vi "measureEcho.vi"() -> ()   [LabVIEW 2016]
uses:
  <vilib>/Utility/file.llb/Write Delimited Spreadsheet (DBL).vi
panel:
  in  "AFC & OFC Measurement time":i32=2
  in  "Burn time/ RFC measurement time":i32=2
  in  "Cluster":T1={"span"=300000000.0, "rbw"=10000.0, "enableVBW"=FALSE, "vbw"=0.0, "traceLength"=64001, "window"=0, "verticalUnit"=0, "center freq"=150000000.0} {"verticalUnit" items=["SpectrumVerticalUnit_dBm", "SpectrumVerticalUnit_Watt", "SpectrumVerticalUnit_Volt", "SpectrumVerticalUnit_Amp", "SpectrumVerticalUnit_dBmV"]; "window" items=["SpectrumWindow_Kaiser", "SpectrumWindow_Mil6dB", "SpectrumWindow_BlackmanHarris", "SpectrumWindow_Rectangle", "SpectrumWindow_FlatTop", "SpectrumWindow_Hann"]; "traceLength" items=["801"=801, "2401"=2401, "4001"=4001, "8001"=8001, "10401"=10401, "16001"=16001, "32001"=32001, "64001"=64001]}
  out "Duration array":T2(array[cluster])
  in  "Array":T3(array[cluster])=[{"Enable ASF?"=TRUE, "Channel Frequency (MHz)"=80.0, "ASF"=0.185, "Enable Frequency Sweep"=FALSE, "Sweep Parameters"={"Start Frequency (MHz)"=80.5, "Stop Frequency (MHz)"=89.25, "Rising Step Size (MHz)"=0.04375, "Falling Step Size (MHz)"=0.0, "Falling Step Interval (ms)"=0.01, "Rising Step Interval (ms)"=1.0}, "Rising/Falling"=FALSE}, {"Enable ASF?"=TRUE, "Channel Frequency (MHz)"=110.0, "ASF"=0.185, "Enable Frequency Sweep"=TRUE, "Sweep Parameters"={"Start Frequency (MHz)"=70.0, "Stop Frequency (MHz)"=160.0, "Rising Step Size (MHz)"=0.0006, "Falling Step Size (MHz)"=0.0, "Falling Step Interval (ms)"=0.01, "Rising Step Interval (ms)"=1.0}, "Rising/Falling"=FALSE}, {"Enable ASF?"=FALSE, "Channel Frequency (MHz)"=80.0, "ASF"=0.1, "Enable Frequency Sweep"=FALSE, "Sweep Parameters"={"Start Frequency (MHz)"=80.5, "Stop Frequency (MHz)"=89.25, "Rising Step Size (MHz)"=0.04375, "Falling Step Size (MHz)"=0.0, "Falling Step Interval (ms)"=0.01, "Rising Step Interval (ms)"=1.0}, "Rising/Falling"=FALSE}, {"Enable ASF?"=TRUE, "Channel Frequency (MHz)"=80.0, "ASF"=0.1, "Enable Frequency Sweep"=TRUE, "Sweep Parameters"={"Start Frequency (MHz)"=40.0, "Stop Frequency (MHz)"=115.0, "Rising Step Size (MHz)"=0.0006, "Falling Step Size (MHz)"=0.0, "Falling Step Interval (ms)"=0.01, "Rising Step Interval (ms)"=1.0}, "Rising/Falling"=FALSE}] {"Sweep Parameters"."Rising Step Interval (ms)" min=0.0 max=2.55 step=0.01 format="%.4f"; "Sweep Parameters"."Stop Frequency (MHz)" min=0.0 max=400.0 step=1.0 format="%.6f"; "Sweep Parameters"."Start Frequency (MHz)" min=0.0 max=400.0 step=1.0 format="%.6f"; "Sweep Parameters"."Falling Step Interval (ms)" min=0.0 max=2.55 step=0.01 format="%.2f"; "Sweep Parameters"."Falling Step Size (MHz)" min=0.0 max=400.0 step=0.1 format="%.6f"; "Sweep Parameters"."Rising Step Size (MHz)" min=0.0 max=400.0 step=0.1 format="%.7f"; "ASF" min=0.0 max=1.0 step=0.001 format="%.3f"; "Channel Frequency (MHz)" min=0.0 max=400.0 step=1.0 format="%.6f"}
  in  "Folder for all data (Don't forget the last slash!)":string="C:\\Users\\Lab\\Desktop\\Data\\2019-08\\2019-08-07\\"
  out "Inst. Freq":dbl=1000000.0
  in  "Shuffle?":bool
  in  "Start freq":dbl=1000000.0 format="%0.2e"
  in  "End freq":dbl=2000000.0 format="%0.2e"
  in  "Freq step":i32=100000 format="%.2e"
  out "error out":errorcluster
  in  "error in":errorcluster
  in  "Mod shape":enum16{"Triangle", "Sine"}(ring)
  # "RSA settings"
  # "Modulation settings"
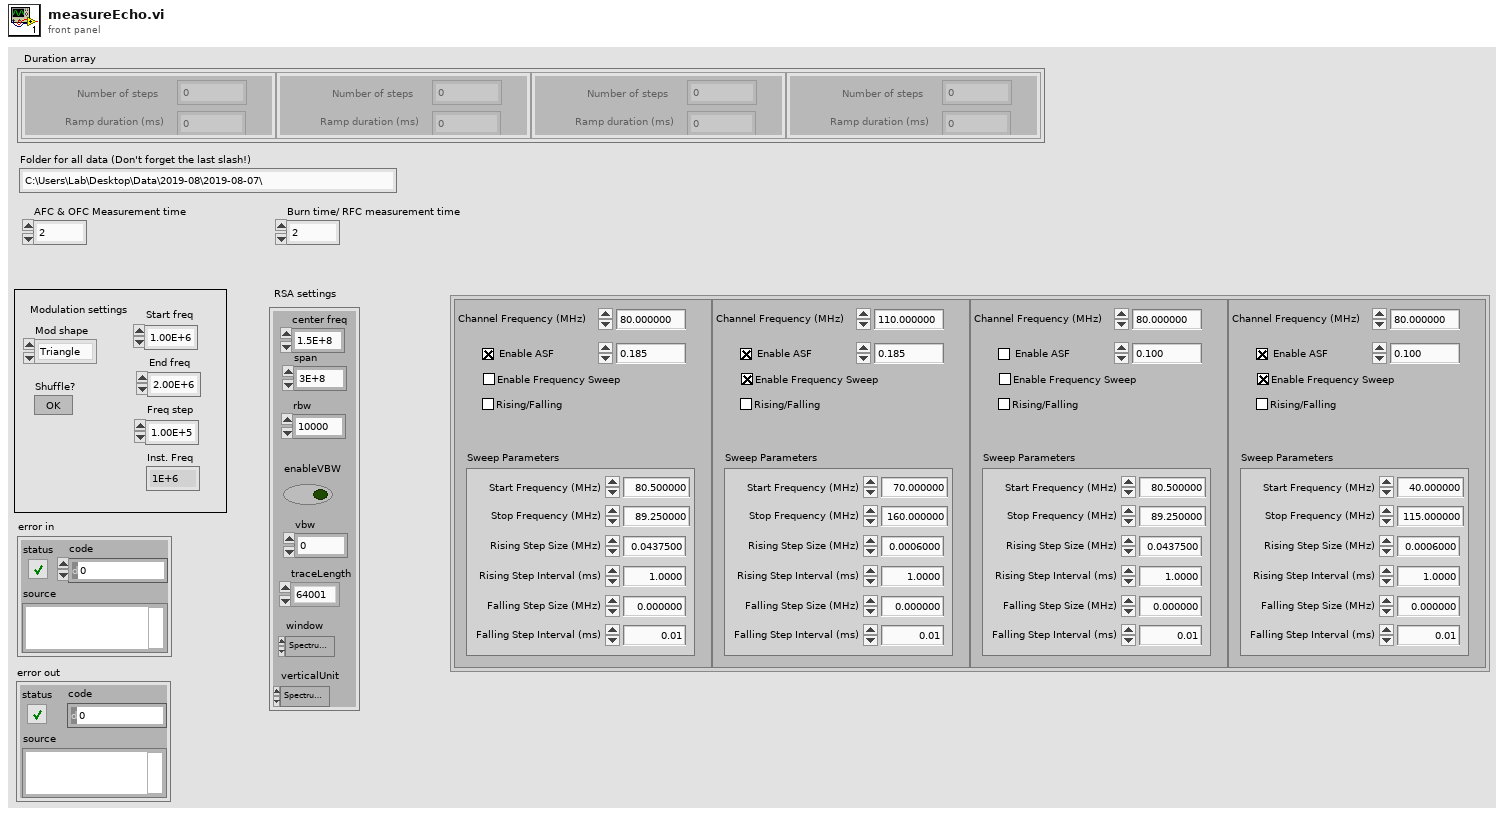
[diagram p1: front panel]
types:
  T1 = cluster{"span":dbl, "rbw":dbl, "enableVBW":bool, "vbw":dbl, "traceLength":u16, "window":u32, "verticalUnit":u32, "center freq":dbl}
  T2 = cluster{"Number of steps":dbl, "Ramp duration (ms)":dbl}[]
  T3 = cluster{"Enable ASF?":bool, "Channel Frequency (MHz)":dbl, "ASF":dbl, "Enable Frequency Sweep":bool, "Sweep Parameters":cluster{"Start Frequency (MHz)":dbl, "Stop Frequency (MHz)":dbl, "Rising Step Size (MHz)":dbl, "Falling Step Size (MHz)":dbl, "Falling Step Interval (ms)":dbl, "Rising Step Interval (ms)":dbl}, "Rising/Falling":bool}[]
  T4 = cluster{"span":dbl, "rbw":dbl, "enableVBW":bool, "vbw":dbl, "traceLength":u16, "window":u32, "verticalUnit":u32}
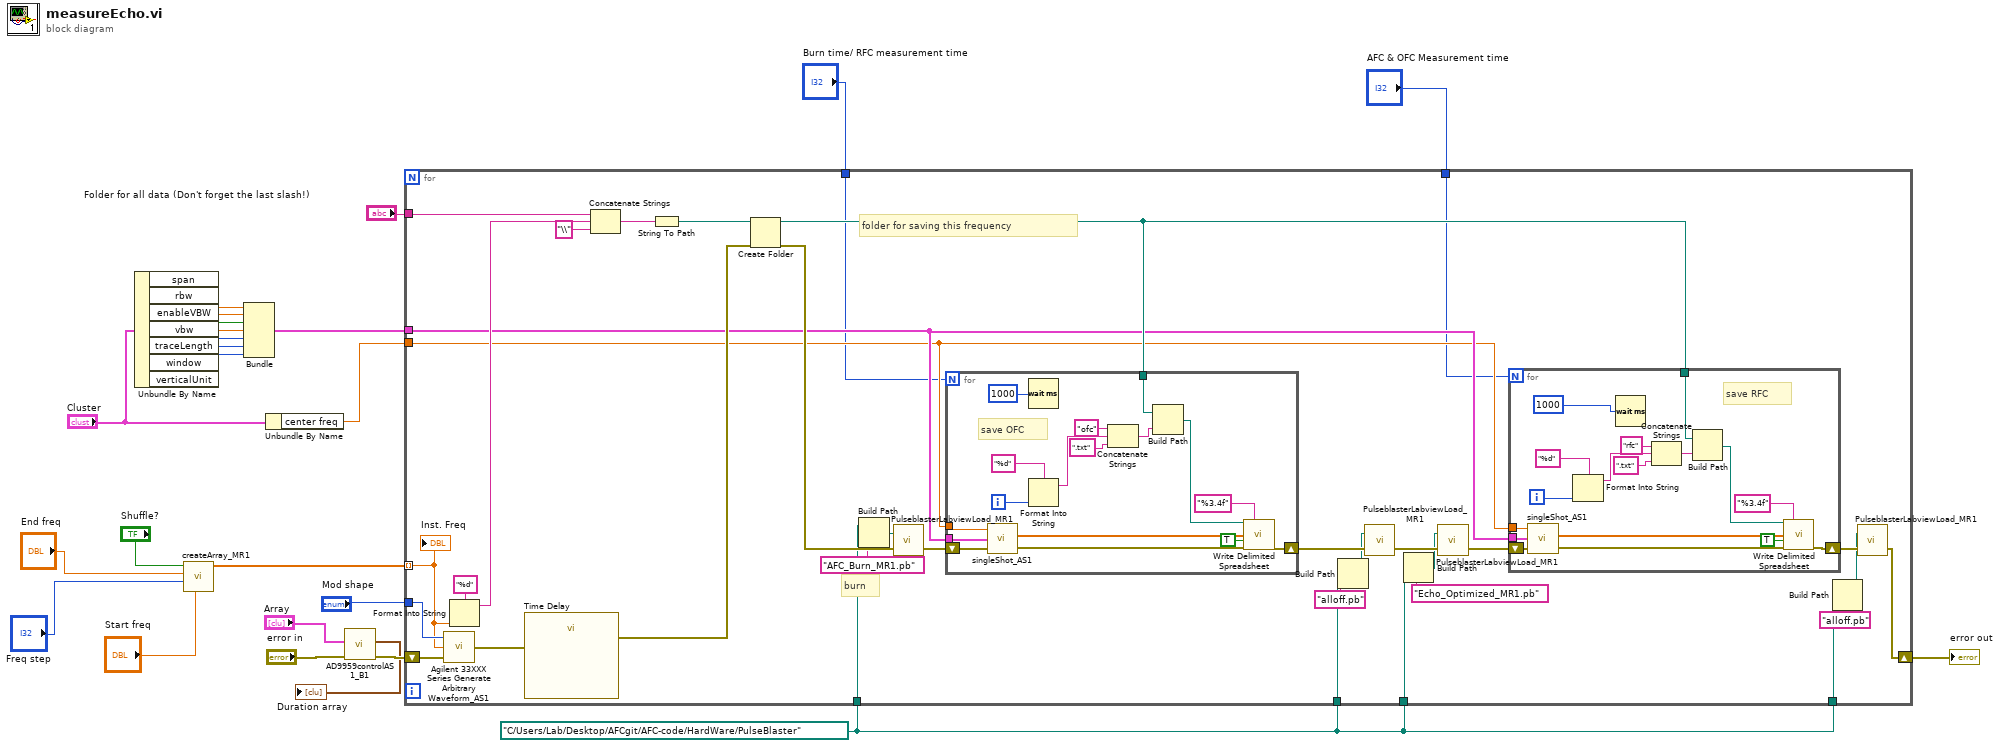
[diagram p0: block diagram]
diagram:
  w22 = path "C:/Users/Lab/Desktop/AFCgit/AFC-code/HardWare/PulseBlaster" ("base path")
  n1 = Unbundle By Name("Cluster") -> ("span"=w10:dbl, "rbw"=w9:dbl, "enableVBW"=w8:bool, "vbw"=w7:dbl, "traceLength"=w6:u16, "window"=w5:u32, "verticalUnit"=w4:u32)
  n2 = call "createArray_MR1.vi"("Start freq"="Start freq", "Freq step"="Freq step", "End freq"="End freq", "Shuffle?"="Shuffle?") -> ("Riffled {X}"=w18:dbl[])  [unwired: 7 in]
  n3 = Bundle("span"=w10, "rbw"=w9, "enableVBW"=w8, "vbw"=w7, "traceLength"=w6, "window"=w5, "verticalUnit"=w4) -> (w3:T4)  [unwired: 1 in]
  n4 = Unbundle By Name("Cluster") -> ("center freq"=w12:dbl)
  n5 = call "AD9959controlAS1_B1.vi"("error in (no error)"="error in", "Array"="Array") -> ("error out"=w19:errorcluster, "Duration array"=→"Duration array":T2)  [unwired: 8 in]
  n6 = for {
    tunnel: w18 -> [w56] mode=indexing
    tunnel: "Mod shape" -> [w60]
    shift-right: [w59] -> w24
    shift-left: w19 -> [w58]
    tunnel: "Folder for all data (Don't forget the last slash!)" -> [w30]
    tunnel: w3 -> [w29]
    tunnel: w22 -> [w41]
    tunnel: w22 -> [w38]
    tunnel: w22 -> [w35]
    tunnel: w22 -> [w32]
    tunnel: w12 -> [w28]
    tunnel: "Burn time/ RFC measurement time" -> [w27]
    tunnel: "AFC & OFC Measurement time" -> [w26]
    # "folder for saving this frequency"
    # "burn"
    n7 = call "Agilent 33XXX Series Generate Arbitrary Waveform_AS1.vi"("error in (no error)"=w58, "Frequency (1000 Hz)"=w56, "Enum"=w60) -> ("error out"=w52:errorcluster)
    n8 = Format Into String(format string="%d", w56) -> (resulting string=w54:string)  [unwired: 2 in, 1 out]
    n9 = call "Time Delay"("error in (no error)"=w52) -> ("error out"=w46:errorcluster)  [unwired: 10 in]
    n10 = Concatenate Strings(w30, w54, "\\" ("string")) -> (w43:string)
    n11 = String To Path(string=w43) -> (path=w42:path)
    n12 = Create Folder(path (use dialog)=w42, error in=w46) -> (created path=w44:path, error out=w45:errorcluster)  [unwired: 1 in, 1 out]
    n13 = Build Path(base path=w41, name or relative path="AFC_Burn_MR1.pb") -> (appended path=w39:path)
    n14 = call "PulseblasterLabviewLoad_MR1.vi"("error in (no error)"=w45, "Input file"=w39) -> ("error out"=w57:errorcluster)  [unwired: 1 out]
    n15 = for {
      N: w27 -> [_]
      shift-right: [w91] -> w48
      shift-left: w57 -> [w94]
      tunnel: w44 -> [w82]
      tunnel: w29 -> [w78]
      tunnel: w28 -> [w79]
      i -> [w80]
      # "save OFC"
      n16 = call "singleShot_AS1.vi"("error in"=w94, "Cluster"=w78, "center freq"=w79) -> ("error out"=w93:errorcluster, "traceData out"=w90:sgl[])
      n17 = Wait (ms)(milliseconds to wait=u32 1000) -> ()  [unwired: 1 out]
      n18 = Format Into String(format string="%d", w80) -> (resulting string=w86:string)  [unwired: 2 in, 1 out]
      n19 = Concatenate Strings("ofc" ("string"), w86, ".txt" ("string")) -> (w85:string)
      n20 = Build Path(base path=w82, name or relative path=w85) -> (appended path=w89:path)
      n21 = call-poly <vilib>:"Write Delimited Spreadsheet.vi"("file path (dialog if empty)"=w89, "format (%.3f)"="%3.4f", "1D data"=w90, "append to file? (new file:F)"=TRUE, "error in (no error)"=w93) -> ("error out"=w91:errorcluster)  [unwired: 9 in, 1 out]
    }
    n22 = Build Path(base path=w35, name or relative path="alloff.pb") -> (appended path=w34:path)
    n23 = call "PulseblasterLabviewLoad_MR1.vi"("error in (no error)"=w48, "Input file"=w34) -> ("error out"=w49:errorcluster)  [unwired: 1 out]
    n24 = Build Path(base path=w38, name or relative path="Echo_Optimized_MR1.pb") -> (appended path=w36:path)
    n25 = call "PulseblasterLabviewLoad_MR1.vi"("error in (no error)"=w49, "Input file"=w36) -> ("error out"=w51:errorcluster)  [unwired: 1 out]
    n26 = for {
      N: w26 -> [_]
      shift-right: [w74] -> w50
      shift-left: w51 -> [w77]
      tunnel: w29 -> [w61]
      tunnel: w44 -> [w64]
      tunnel: w28 -> [w62]
      i -> [w69]
      # "save RFC"
      n27 = call "singleShot_AS1.vi"("error in"=w77, "Cluster"=w61, "center freq"=w62) -> ("error out"=w76:errorcluster, "traceData out"=w73:sgl[])
      n28 = Format Into String(format string="%d", w69) -> (resulting string=w68:string)  [unwired: 2 in, 1 out]
      n29 = Wait (ms)(milliseconds to wait=u32 1000) -> ()  [unwired: 1 out]
      n30 = Concatenate Strings("rfc" ("string"), w68, ".txt" ("string")) -> (w67:string)
      n31 = Build Path(base path=w64, name or relative path=w67) -> (appended path=w72:path)
      n32 = call-poly <vilib>:"Write Delimited Spreadsheet.vi"("file path (dialog if empty)"=w72, "format (%.3f)"="%3.4f", "1D data"=w73, "append to file? (new file:F)"=TRUE, "error in (no error)"=w76) -> ("error out"=w74:errorcluster)  [unwired: 9 in, 1 out]
    }
    n33 = Build Path(base path=w32, name or relative path="alloff.pb") -> (appended path=w31:path)
    n34 = call "PulseblasterLabviewLoad_MR1.vi"("error in (no error)"=w50, "Input file"=w31) -> ("error out"=w59:errorcluster)  [unwired: 1 out]
    "Inst. Freq" <- w56
  }
  "error out" <- w24
